vi "RT - Analog Signals.vi"(6 "Send AI Alarms?":bool, 8 "error in":errorcluster, 10 "Analog In":refnum<k21>[](array[refnum]), 11 "Message Queue":refnum<queue>) -> (0 "error out":errorcluster, 2 "Analog Signals":dbl[](array[numeric]), 3 "dup Message Queue":refnum<queue>)   [LabVIEW 2018]
uses:
  Message Queue/Message Cluster.ctl
  Message Queue/Message.ctl
  Message Queue/Message Queue.lvlib
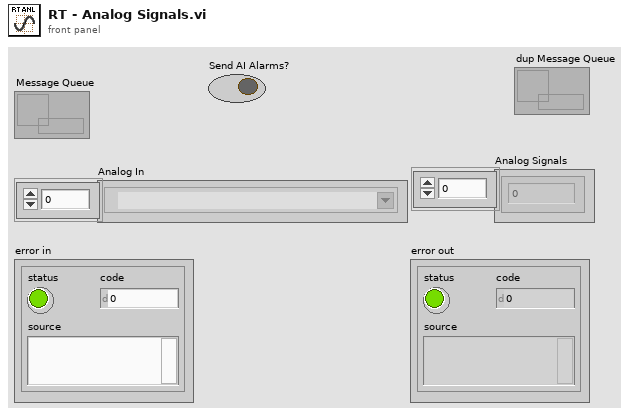
[diagram p1: front panel]
types:
  T1 = typedef "Message Queue.lvlib/Message.ctl" = enum16{"Initialize", "Initialize UI Refs", "Disable Controls", "Enable UI Controls", "Connect RT", "Get Control Mode from RT", "Send Control Mode to UI", "Update Control Mode", "Get Config from RT", "Send Config to UI", "Update Parameters", "Change Parameters", "Calibrate Config", "Update Calibration", "Change Valve State", "Get Valve Status from RT", "Send Valve Status to UI", "Update Valve Status", "Inital UI Values", "Disconnect RT", "Close Connection", "Disconnect UI", "Run Mode", "Stop ALL", "Change Control Mode", "Skid Manual", "Computer Manual", "Step Automated", "Fully Automated", "Reset", "Pumps Command", "Pump State Changed", "Critical Error", "Log-Only Error", "Non-Critical Error", "RT Error", "Update System Status", "Update DI Status", "Clear System Status", "Update Warning", "Clear Warning", "Upate Timeout", "Update Reset Status", "Waiting", "Verify Password", "Manual Cleaning Process", "Update Manual Cleaning Process", "Cal - Body", "Cal - US", "Cal - Update Parameters", "AddSub - BleedValve", "AddSub - TCValve", "AddSub - ABValve", "AddSub - TriplexPump", "Propotional Update", "Exit", "---Copy This Frame---"}
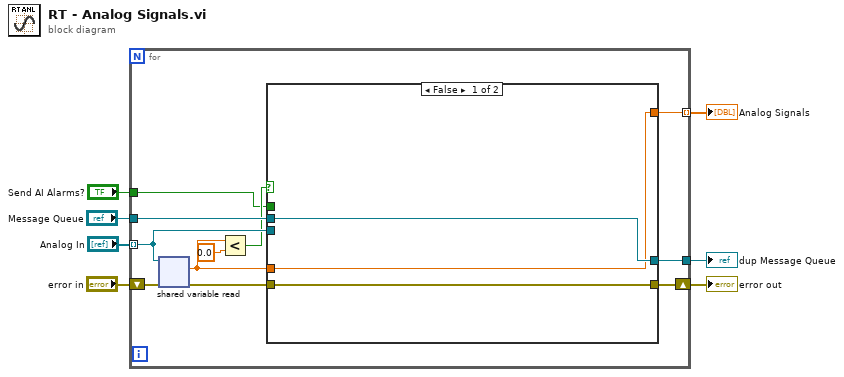
[diagram p0: block diagram]
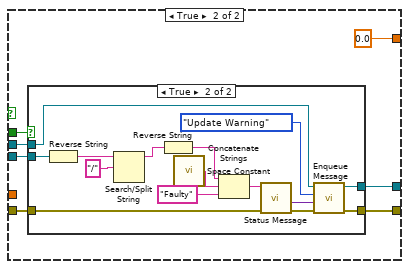
[diagram p2: hidden frame]
diagram:
  n1 = for {
    tunnel: [w15] -> w1 mode=indexing
    tunnel: "Analog In" -> [w10] mode=indexing
    shift-right: [w13] -> w2
    shift-left: "error in" -> [w18]
    tunnel: "Message Queue" -> [w17]
    tunnel: [w16] -> w4
    tunnel: "Send AI Alarms?" -> [w8]
    n2 = shared-variable-read(w10, w18) -> (w14:errorcluster, w12:dbl)  [unwired: 2 out]
    n3 = Less?(x=w12, y=0.0) -> (x < y?=w9:bool)
    n4 = case shown="False" w9 {
      tunnel: w17 -> [w21 w28]
      tunnel: [w21 w27] -> w16
      tunnel: w12 -> [w19 _]
      tunnel: [w19 0.0] -> w15
      tunnel: w14 -> [w20 w24]
      tunnel: [w20 w26] -> w13
      tunnel: w10 -> [_ w25]
      tunnel: w8 -> [_ w22]
      frame False {
      }
      frame True {
        n5 = case shown="True" w22 {
          tunnel: w28 -> [w30 w45]
          tunnel: [w30 w44] -> w27
          tunnel: [w29 w43] -> w26
          tunnel: w25 -> [_ w38]
          tunnel: w24 -> [w29 w36]
          frame False {
          }
          frame True {
            n6 = Reverse String(1:w38) -> (0:w39:string)
            n7 = Search/Split String(string=w39, search string/char (-)="/") -> (substring before match=w41:string)  [unwired: 1 in, 2 out]
            n8 = Reverse String(1:w41) -> (0:w34:string)
            n9 = call <vilib>:"Space Constant.vi"() -> ("String"=w33:string)
            n10 = Concatenate Strings(w34, w33, "Faulty" ("string")) -> (w31:string)
            n11 = call "Status Message.vi"("Error In"=w36, "Message"=w31) -> ("Error Out"=w35:errorcluster, "Status"=w37:variant)  [unwired: 7 in]
            n12 = call "Enqueue Message.vi"("error in (no error)"=w35, "Message Data"=w37, "Message"=Message."Update Warning", "Message Queue"=w45) -> ("error out"=w43:errorcluster, "dup Message Queue"=w44:refnum<queue>)  [unwired: 6 in]
          }
        }
      }
    }
  }
  "error out" <- w2
  "dup Message Queue" <- w4
  "Analog Signals" <- w1
